vi "Filter_update.vi"(0 "new coeffs":bool, 1 "new shift":i32, 2 "new coeffs":fxp<+/-,18,18>[](array[numeric]), 3 "config rdy for data":bool, 5 "reload rdy for data":bool) -> (10 "busy":bool, 11 "s_axis_reload_tlast":bool, 14 "s_axis_config_tvalid":bool, 15 "shift out":i32, 16 "s_axis_config_tdata":fxp<+,8,8>, 17 "s_axis_reload_tvalid":bool, 19 "s_axis_reload_tdata":fxp<+,24,24>)   [LabVIEW 2013]
uses:
  <vilib>/rvi/FXPMathLib/FxpConvert/subVIs/nifxpmath_Convert_SimConfig.ctl
  <vilib>/fxp/LVFixedPointQuantizationPolicyTypeDef.ctl
  <vilib>/fxp/LVFixedPointOverflowPolicyTypeDef.ctl
  <vilib>/rvi/FXPMathLib/FxpConvert/simVIs/DllFxpConvertTemp_sub.vi
  <vilib>/rvi/FXPMathLib/FxpConvert/XNode/nifxpmath_Convert.xnode
  <vilib>/rvi/FXPMathLib/FxpAdd/XNode/nifxpmath_Add.xnode
  <vilib>/rvi/FXPMathLib/FxpInterpret/XNode/nifxpmath_Interpret.xnode
  <vilib>/rvi/FXPMathLib/sim/FxpSim.dll
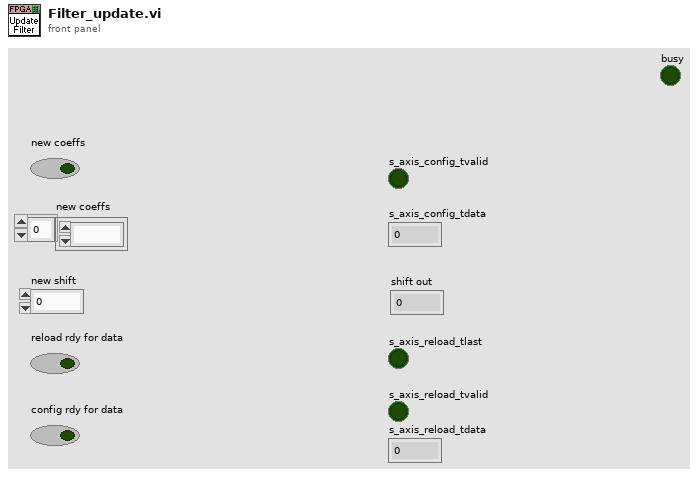
[diagram p1: front panel]
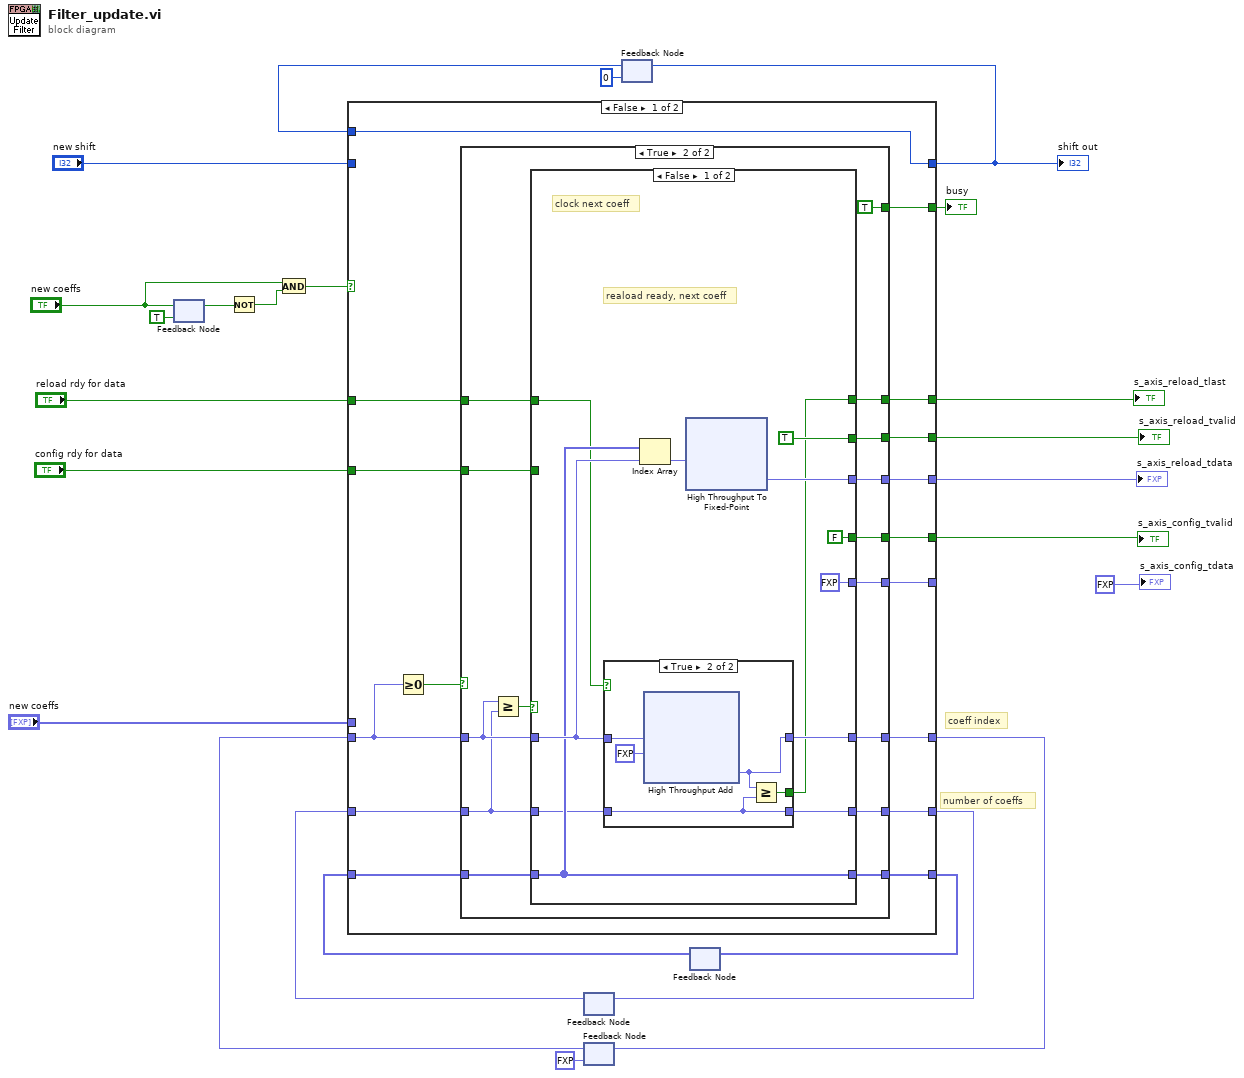
[diagram p0: block diagram]
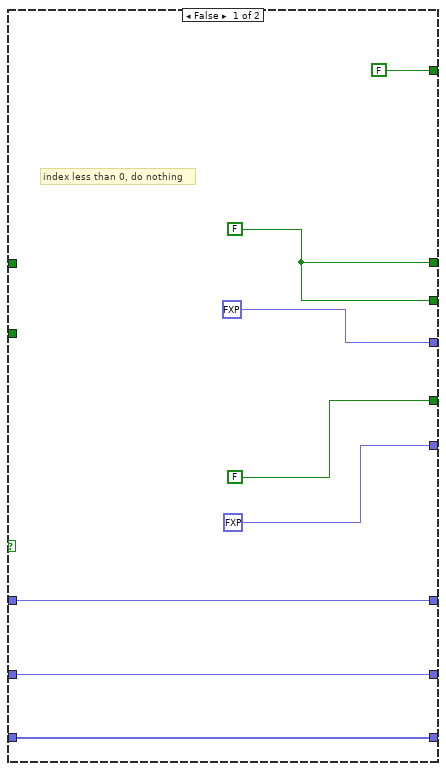
[diagram p2: hidden frame]
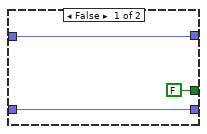
[diagram p3: hidden frame]
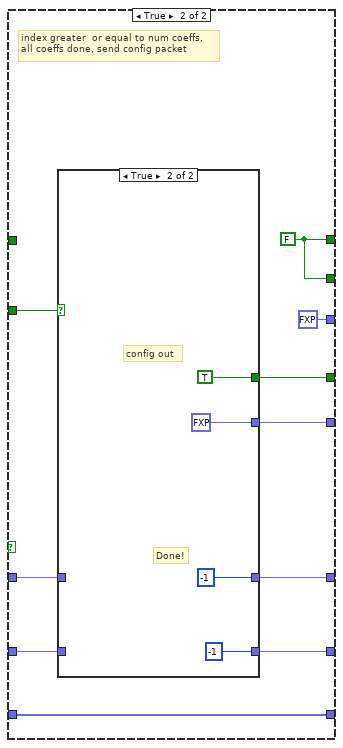
[diagram p4: hidden frame]
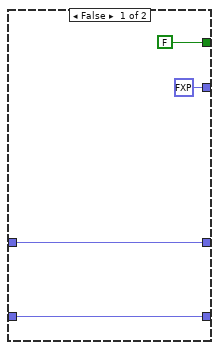
[diagram p5: hidden frame]
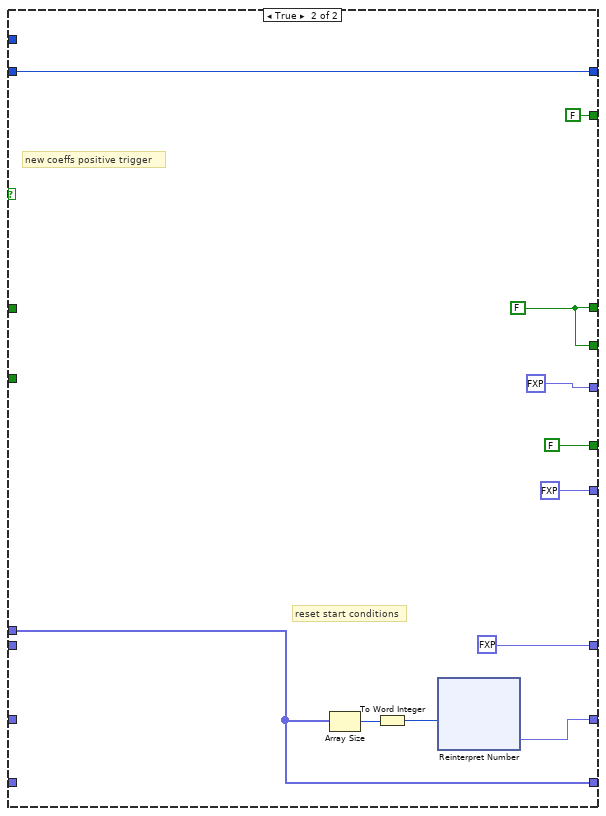
[diagram p6: hidden frame]
diagram:
  # "number of coeffs"
  # "coeff index"
  n1 = feedback-in #1("new coeffs") -> ()
  n2 = feedback #1(TRUE ("new coeffs")) -> (w25:bool)
  n3 = Not(x=w25) -> (.not. x?=w24:bool)
  n4 = And(x="new coeffs", y=w24) -> (x .and. y?=w22:bool)
  n5 = feedback #2() -> (w13:fxp<+/-,16,16>)  [unwired: 1 in]
  n6 = feedback #3(fxp<+/-,16,16> -1.0 ("s_axis_reload_tdata 2")) -> (w5:fxp<+/-,16,16>)
  n7 = feedback #4(0 ("new shift")) -> (w2:i32)
  n8 = feedback #5() -> (w19:fxp<+/-,18,18>[])  [unwired: 1 in]
  n9 = case shown="False" w22 {
    tunnel: "new coeffs" -> [_ w133]
    tunnel: [w38 w133] -> w20
    tunnel: w19 -> [w37 _]
    tunnel: [w39 fxp<+/-,16,16> 0.0 ("s_axis_reload_tdata 2")] -> w18
    tunnel: w5 -> [w40 _]
    tunnel: [w34 w135] -> w17
    tunnel: [w33 w135] -> w16
    tunnel: [w32 fxp<+,24,24> 0.0 ("s_axis_reload_tdata")] -> w15
    tunnel: [w36 w127] -> w14
    tunnel: w13 -> [w35 _]
    tunnel: [w31 FALSE] -> w12
    tunnel: [w30 fxp<+,8,8> 0.0 ("s_axis_config_tdata")] -> _
    tunnel: "reload rdy for data" -> [w29 _]
    tunnel: "config rdy for data" -> [w28 _]
    tunnel: [w27 FALSE] -> w7
    tunnel: [w26 w125] -> w3
    tunnel: "new shift" -> [_ w125]
    tunnel: w2 -> [w26 _]
    frame False {
      n10 = Greater Or Equal To 0?(x=w40) -> (x >= 0?=w41:bool)
      n11 = case shown="True" w41 {
        tunnel: w40 -> [w49 w63]
        tunnel: [w49 w57] -> w39
        tunnel: [w48 w56] -> w38
        tunnel: w37 -> [w48 w64]
        tunnel: [w47 w55] -> w36
        tunnel: w35 -> [w47 w61]
        tunnel: [w46 w51] -> w34
        tunnel: [w46 w52] -> w33
        tunnel: [fxp<+,24,24> 0.0 ("s_axis_reload_tdata") w53] -> w32
        tunnel: [FALSE w59] -> w31
        tunnel: [fxp<+,8,8> 0.0 ("s_axis_config_tdata") w58] -> w30
        tunnel: w29 -> [_ w54]
        tunnel: w28 -> [_ w60]
        tunnel: [FALSE TRUE] -> w27
        frame False {
          w46 = FALSE
          # "index less than 0, do nothing"
        }
        frame True {
          n12 = Greater Or Equal?(x=w63, y=w61) -> (x >= y?=w62:bool)
          n13 = case shown="False" w62 {
            tunnel: w64 -> [w74 w112]
            tunnel: w63 -> [w76 w110]
            tunnel: w61 -> [w71 w109]
            tunnel: w60 -> [_ w116]
            tunnel: [FALSE w115] -> w59
            tunnel: [fxp<+,8,8> 0.0 ("s_axis_config_tdata") w114] -> w58
            tunnel: [w73 w113] -> w57
            tunnel: [w74 w112] -> w56
            tunnel: [w65 w111] -> w55
            tunnel: w54 -> [w66 _]
            tunnel: [w75 fxp<+,24,24> 0.0 ("y")] -> w53
            tunnel: [TRUE w108] -> w52
            tunnel: [w70 w108] -> w51
            frame False {
              # "reaload ready, next coeff"
              # "clock next coeff"
              n14 = case shown="True" w66 {
                tunnel: w76 -> [w79 w84]
                tunnel: [w79 w83] -> w73
                tunnel: w71 -> [w77 w80]
                tunnel: [FALSE w82] -> w70
                tunnel: [w77 w80] -> w65
                frame False {
                }
                frame True {
                  n15 = xnode "High Throughput Add"("x"=w84, "y"=fxp<+/-,16,16> 1.0) -> ("x+y"=w83:fxp<+/-,16,16>)
                  n16 = Greater Or Equal?(x=w83, y=w80) -> (x >= y?=w82:bool)
                }
              }
              n17 = Index Array(array=w74, index=w76) -> (element=w67:fxp<+/-,18,18>)
              n18 = xnode "High Throughput To Fixed-Point"("x"=w67) -> ("y"=w75:fxp<+,24,24>)
            }
            frame True {
              w108 = FALSE
              # "index greater  or equal to num coeffs,\nall coeffs done, send config packet"
              n19 = case shown="True" w116 {
                tunnel: [FALSE TRUE] -> w115
                tunnel: [fxp<+,8,8> 0.0 ("s_axis_config_tdata") fxp<+,8,8> 0.0 ("s_axis_config_tdata")] -> w114
                tunnel: [w119 i16 -1] -> w113
                tunnel: [w118 i16 -1] -> w111
                tunnel: w110 -> [w119 _]
                tunnel: w109 -> [w118 _]
                frame False {
                }
                frame True {
                  # "Done!"
                  # "config out"
                }
              }
            }
          }
        }
      }
    }
    frame True {
      w135 = FALSE
      # "reset start conditions"
      # "new coeffs positive trigger"
      n20 = Array Size(array=w133) -> (size(s)=w132:i32)
      n21 = To Word Integer(number=w132) -> (16bit integer=w128:i16)
      n22 = xnode "Reinterpret Number"("x"=w128) -> ("y"=w127:fxp<+/-,16,16>)
    }
  }
  "s_axis_reload_tdata" <- w15
  "s_axis_config_tvalid" <- w12
  "s_axis_reload_tvalid" <- w16
  "s_axis_reload_tlast" <- w17
  "busy" <- w7
  "shift out" <- w3
  n23 = feedback-in #2(w14) -> ()
  n24 = feedback-in #3(w18) -> ()
  n25 = feedback-in #4(w3) -> ()
  n26 = feedback-in #5(w20) -> ()
  "s_axis_config_tdata" <- fxp<+,8,8> 0.0 ("s_axis_config_tdata")
